vi "例程35-数字FIR滤波器的使用.vi"() -> ()   [LabVIEW 2016]
uses:
  <vilib>/measure/macond.llb/FIR Filter for N Chan.vi
  <vilib>/measure/NI_MAPro.lvlib
panel:
  out "波形图 2":waveform(dbl)[](graph)
  out "波形图":dynamicdata(graph)
  out "signal(s) out":waveform(dbl)[](array[waveform]) caption="信号输出"
  out "filter information":T1 caption="滤波器信息" {"phase H(w)"."df" format="%.2p"; "phase H(w)"."f0" format="%.2p"; "phase H(w)"."Phase H(w)" format="%.2p"; "magnitude H(w)"."df" format="%.2p"; "magnitude H(w)"."f0" format="%.2p"; "magnitude H(w)"."Mag H(w)" format="%.2p"}
  out "error out 2":errorcluster caption="错误输出"
  in  "error in (no error) 2":errorcluster caption="错误输入（无错误）"
  in  "reset filters":bool caption="重置滤波器"
  in  "FIR filter specifications":T2={"Topology"=enum."Off", "Type"=enum."Lowpass", "#Taps"=50, "Lower PB"=100.0, "Upper PB"=0.0, "Lower SB"=200.0, "Upper SB"=0.0} caption="FIR滤波器规范" {"Lower SB" format="%0.2p"; "Upper SB" format="%0.2p"; "Lower PB" format="%0.2p"; "Upper PB" format="%0.2p"}
  in  "optional FIR filter specifications":T3={"PB Gain"=-3.0, "SB Gain"=-60.0, "Scale"=TRUE, "Window"=enum."Flat Top"} caption="可选FIR滤波器规范" {"SB Gain" format="%.2p"; "PB Gain" format="%.2p"}
  out "error out":errorcluster caption="错误输出"
  in  "Seed Number":dbl=-1.0 caption="种子值"
  in  "噪声幅值":dbl=0.6
  in  "error in (no error)":errorcluster caption="错误输入（无错误）"
  in  "Phase":dbl caption="相位"
  in  "Amplitude":dbl=1.0 caption="幅值"
  in  "Frequency":dbl=10.1 caption="频率"
  in  "Reset Signal":bool caption="重置信号"
  in  "Offset":dbl caption="偏移量"
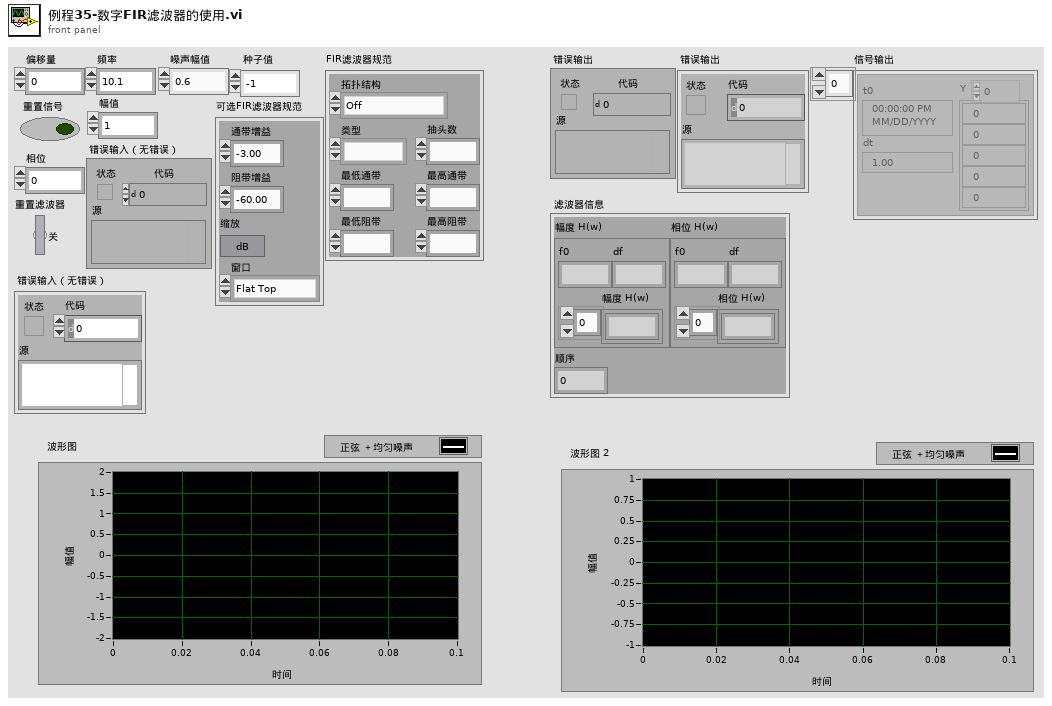
[diagram p1: front panel]
types:
  T1 = cluster{"magnitude H(w)":cluster{"f0":dbl, "df":dbl, "Mag H(w)":dbl[]}, "phase H(w)":cluster{"f0":dbl, "df":dbl, "Phase H(w)":dbl[]}, "order":i32}
  T2 = cluster{"Topology":enum16{"Off", "FIR by Specification", "Equi-ripple FIR", "Windowed FIR"}, "Type":enum16{"Lowpass", "Highpass", "Bandpass", "Bandstop"}, "#Taps":i32, "Lower PB":dbl, "Upper PB":dbl, "Lower SB":dbl, "Upper SB":dbl}
  T3 = cluster{"PB Gain":dbl, "SB Gain":dbl, "Scale":bool, "Window":enum16{"None", "Hanning", "Hamming", "Triangular", "Blackman", "Exact Blackman", "Blackman-Harris", "Kaiser-Bessel", "Flat Top"}}
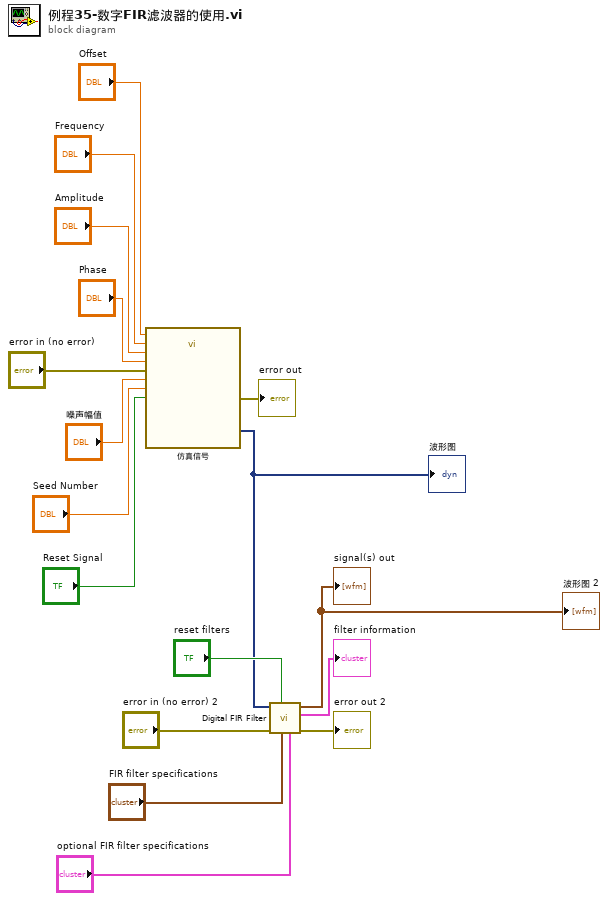
[diagram p0: block diagram]
diagram:
  n1 = call "仿真信号"("Offset"="Offset", "Reset Signal"="Reset Signal", "Frequency"="Frequency", "Amplitude"="Amplitude", "Phase"="Phase", "error in (no error)"="error in (no error)", "噪声幅值"="噪声幅值", "Seed Number"="Seed Number") -> ("正弦与均匀噪声"=w2:dynamicdata, "error out"=→"error out":errorcluster)  [unwired: 6 in]
  "波形图" <- w2
  n2 = call-poly <vilib>:"Digital FIR Filter.vi"("optional FIR filter specifications"="optional FIR filter specifications", "FIR filter specifications"="FIR filter specifications", "reset filters"="reset filters", "error in (no error)"="error in (no error) 2", "signal(s) in"=w2) -> ("error out"=→"error out 2":errorcluster, "filter information"=→"filter information":T1, "signal(s) out"=→"signal(s) out" →"波形图 2":waveform(dbl)[])  [unwired: 4 in]
